vi "CreateFile.vi"(11 "date/time string":string) -> (3 "appended path":path)   [LabVIEW 2026]
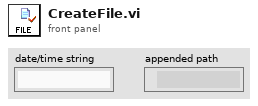
[diagram p1: front panel]
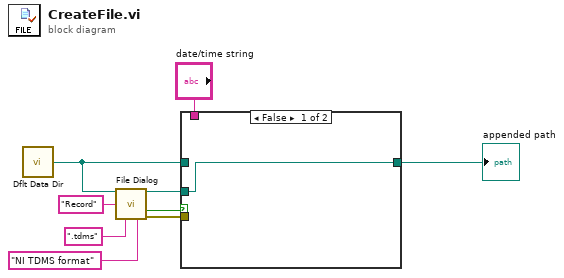
[diagram p0: block diagram]
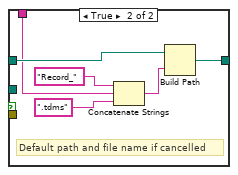
[diagram p2: hidden frame]
diagram:
  n1 = call <vilib>:"Dflt Data Dir.vi"() -> ("App:Default Data Directory"=w6:path)
  n2 = call "File Dialog"("start path"=w6, "default name"="Record", "pattern (all files)"=".tdms", "pattern label"="NI TDMS format") -> ("selected path"=w1:path, "cancelled"=w5:bool, "error out"=w7:errorcluster)  [unwired: 8 in, 1 out]
  n3 = case shown="False" w5 {
    tunnel: w6 -> [_ w14]
    tunnel: [w10 w12] -> w9
    tunnel: w7 -> [_ _]
    tunnel: "date/time string" -> [_ w11]
    tunnel: w1 -> [w10 _]
    frame False {
    }
    frame True {
      # "Default path and file name if cancelled"
      n4 = Concatenate Strings("Record_", w11, ".tdms" ("string")) -> (w13:string)
      n5 = Build Path(base path=w14, name or relative path=w13) -> (appended path=w12:path)
    }
  }
  "appended path" <- w9
